vi "IRSafety.vi"(1 "MillisecondsBetweenThreshold":dbl=500.0, 2 "threshold":dbl=0.05, 3 "VoltageWhenUnplugged":dbl=0.24, 4 "Voltage":dbl) -> (0 "Boolean":bool)   [LabVIEW 2019]
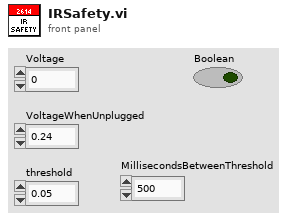
[diagram p1: front panel]
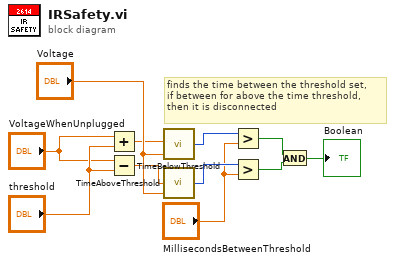
[diagram p0: block diagram]
diagram:
  # "finds the time between the threshold set, \nif between for above the time threshold,\nthen it is disconnected"
  n1 = Add(x="VoltageWhenUnplugged", y="threshold") -> (x+y=w7:dbl)
  n2 = Subtract(x="VoltageWhenUnplugged", y="threshold") -> (x-y=w8:dbl)
  n3 = call "TimeBelowThreshold.vi"("Current Value"="Voltage", "Threshold"=w7) -> ("Time Below"=w10:u32)  [unwired: 3 in]
  n4 = call "TimeAboveThreshold.vi"("Current Value"="Voltage", "Threshold"=w8) -> ("Time Above"=w11:u32)  [unwired: 3 in]
  n5 = Greater?(x=w10, y="MillisecondsBetweenThreshold") -> (0:w3:bool)
  n6 = Greater?(x=w11, y="MillisecondsBetweenThreshold") -> (0:w4:bool)
  n7 = And(x=w3, y=w4) -> (x .and. y?=→"Boolean":bool)
